vi "Motors Move Speed.vi"(7 "Speed (mm or degree/sec)":dbl, 8 "error in":errorcluster, 9 "VISA in":refnum<visa-resource-name>, 10 "Axis":u32=1, 11 "Axis Multiplier":u32) -> (0 "error out":errorcluster, 1 "VISA out":refnum<visa-resource-name>)   [LabVIEW 2018]
panel:
  out "Read Buffer":string
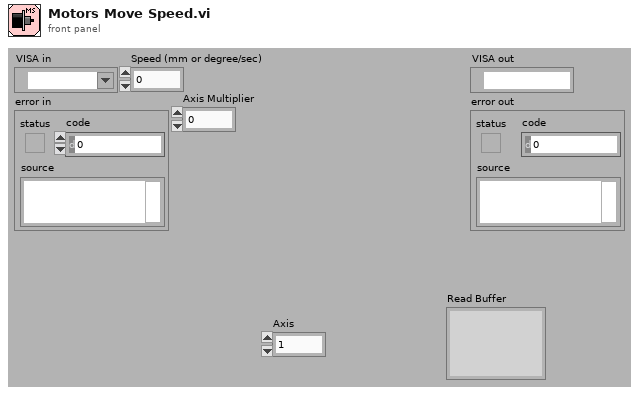
[diagram p1: front panel]
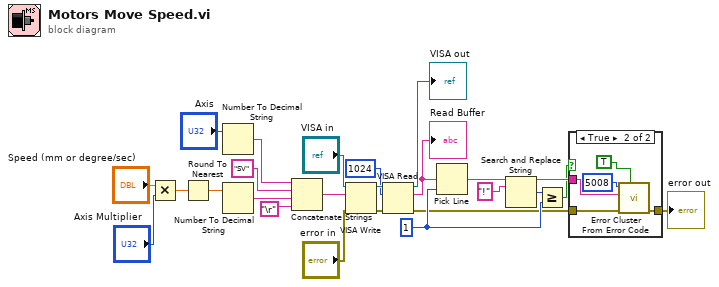
[diagram p0: block diagram]
diagram:
  w10 = 1 ("line index")
  n1 = Multiply(x="Speed (mm or degree/sec)", y="Axis Multiplier") -> (x*y=w7:dbl)
  n2 = Round To Nearest(number=w7) -> (nearest integer value=w6:dbl)
  n3 = Number To Decimal String(number="Axis") -> (decimal integer string=w13:string)  [unwired: 1 in]
  n4 = Number To Decimal String(number=w6) -> (decimal integer string=w19:string)  [unwired: 1 in]
  n5 = Concatenate Strings(w13, "SV" ("Command"), w19, "\r") -> (w20:string)
  n6 = VISA Write(VISA resource name="VISA in", write buffer=w20, error in (no error)="error in") -> (VISA resource name out=w23:refnum<visa-resource-name>, error out=w24:errorcluster)  [unwired: 1 out]
  n7 = VISA Read(VISA resource name=w23, byte count=1024, error in (no error)=w24) -> (VISA resource name out=→"VISA out":refnum<visa-resource-name>, read buffer=w16:string, error out=w1:errorcluster)  [unwired: 1 out]
  "Read Buffer" <- w16
  n8 = Pick Line(multi-line string=w16, line index=w10) -> (output string=w15:string)  [unwired: 1 in]
  n9 = Search and Replace String(input string=w15, search string="!") -> (result string=w14:string, number of replacements=w17:i32)  [unwired: 6 in, 2 out]
  n10 = Greater Or Equal?(x=w17, y=w10) -> (x >= y?=w4:bool)
  n11 = case shown="True" w4 {
    tunnel: w14 -> [_ w28]
    tunnel: [w26 w30] -> w2
    tunnel: w1 -> [w26 w31]
    frame False {
    }
    frame True {
      n12 = call <vilib>:"Error Cluster From Error Code.vi"("show call chain? (False)"=TRUE, "error in (no error)"=w31, "error message (\"\")"=w28, "error code (0)"=5008) -> ("error out"=w30:errorcluster)  [unwired: 5 in]
    }
  }
  "error out" <- w2
